vi "myRIO_BRig_FPGA_v3,50.vi"() -> ()   [LabVIEW 2014]
uses:
  <vilib>/rvi/FXPMathLib/FxpMul/XNode/nifxpmath_Multiplier.xnode
  <vilib>/rvi/FXPMathLib/sim/FxpSim.dll
  <vilib>/eio/EIONode/EIONode.xnode
  <vilib>/rvi/eio/common/nirviEmuTemplateMethod_errors.vi
panel:
  in  "k1__counter_per_ms":u16=100 min=100 max=40000 step=1
  in  "laser_Nshutter":u32=100
  in  "AnaOut_0":u16
  in  "laser_Nvalley":u32=100
  in  "laser_Npeak":u32=100
  in  "laserledMTrig":bool
  in  "laser_selWro_Ntotal":u32=100
  in  "laser_selWro_NDelay":u32
  in  "laser_selRew_Ntotal":u32=100
  in  "laser_selRew_Ndelay":u32
  in  "laserResponse_reward_LED":bool
  in  "laserResponse_wrong_LED":bool
  out "SelectWrong":bool
  out "SelectReward":bool
  in  "laserResponse_wrong":bool
  in  "laserResponse_reward":bool
  in  "Left(F)_or_Right(T)":bool
  in  "ignoreWrong":bool
  in  "SelectionState":bool
  in  "laserMTrig":bool
  in  "FPGA_Stop":bool
  in  "audioTrigger_L":bool
  in  "audioTrigger_R":bool
  in  "audioFreq_L_kHz":u8=14 min=1 max=14 step=1
  in  "audioAmp_L":u16=1 min=1 max=32767 step=1
  in  "audioFreq_R_kHz":u8=14 min=1 max=14 step=1
  in  "audioAmp_R":u16=1 min=1 max=32767 step=1
  in  "A3_SL":bool
  in  "A1_SR":bool
  in  "Counts_Reset":bool
  out "A4_LickR":u32
  out "A2_LickL":u32
  in  "A6_Act":bool
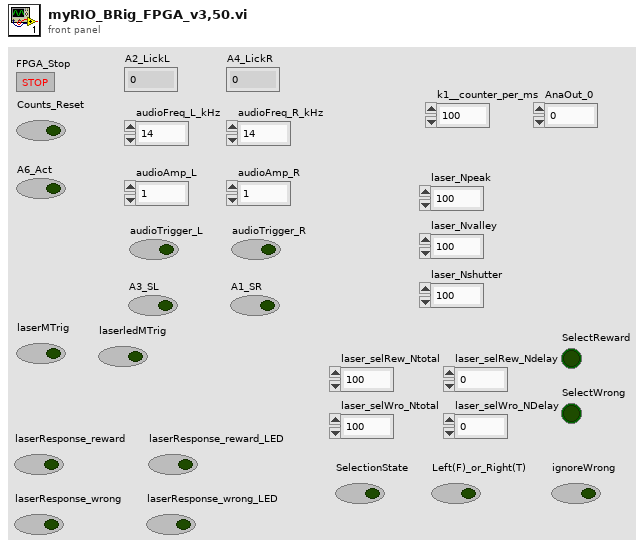
[diagram p1: front panel]
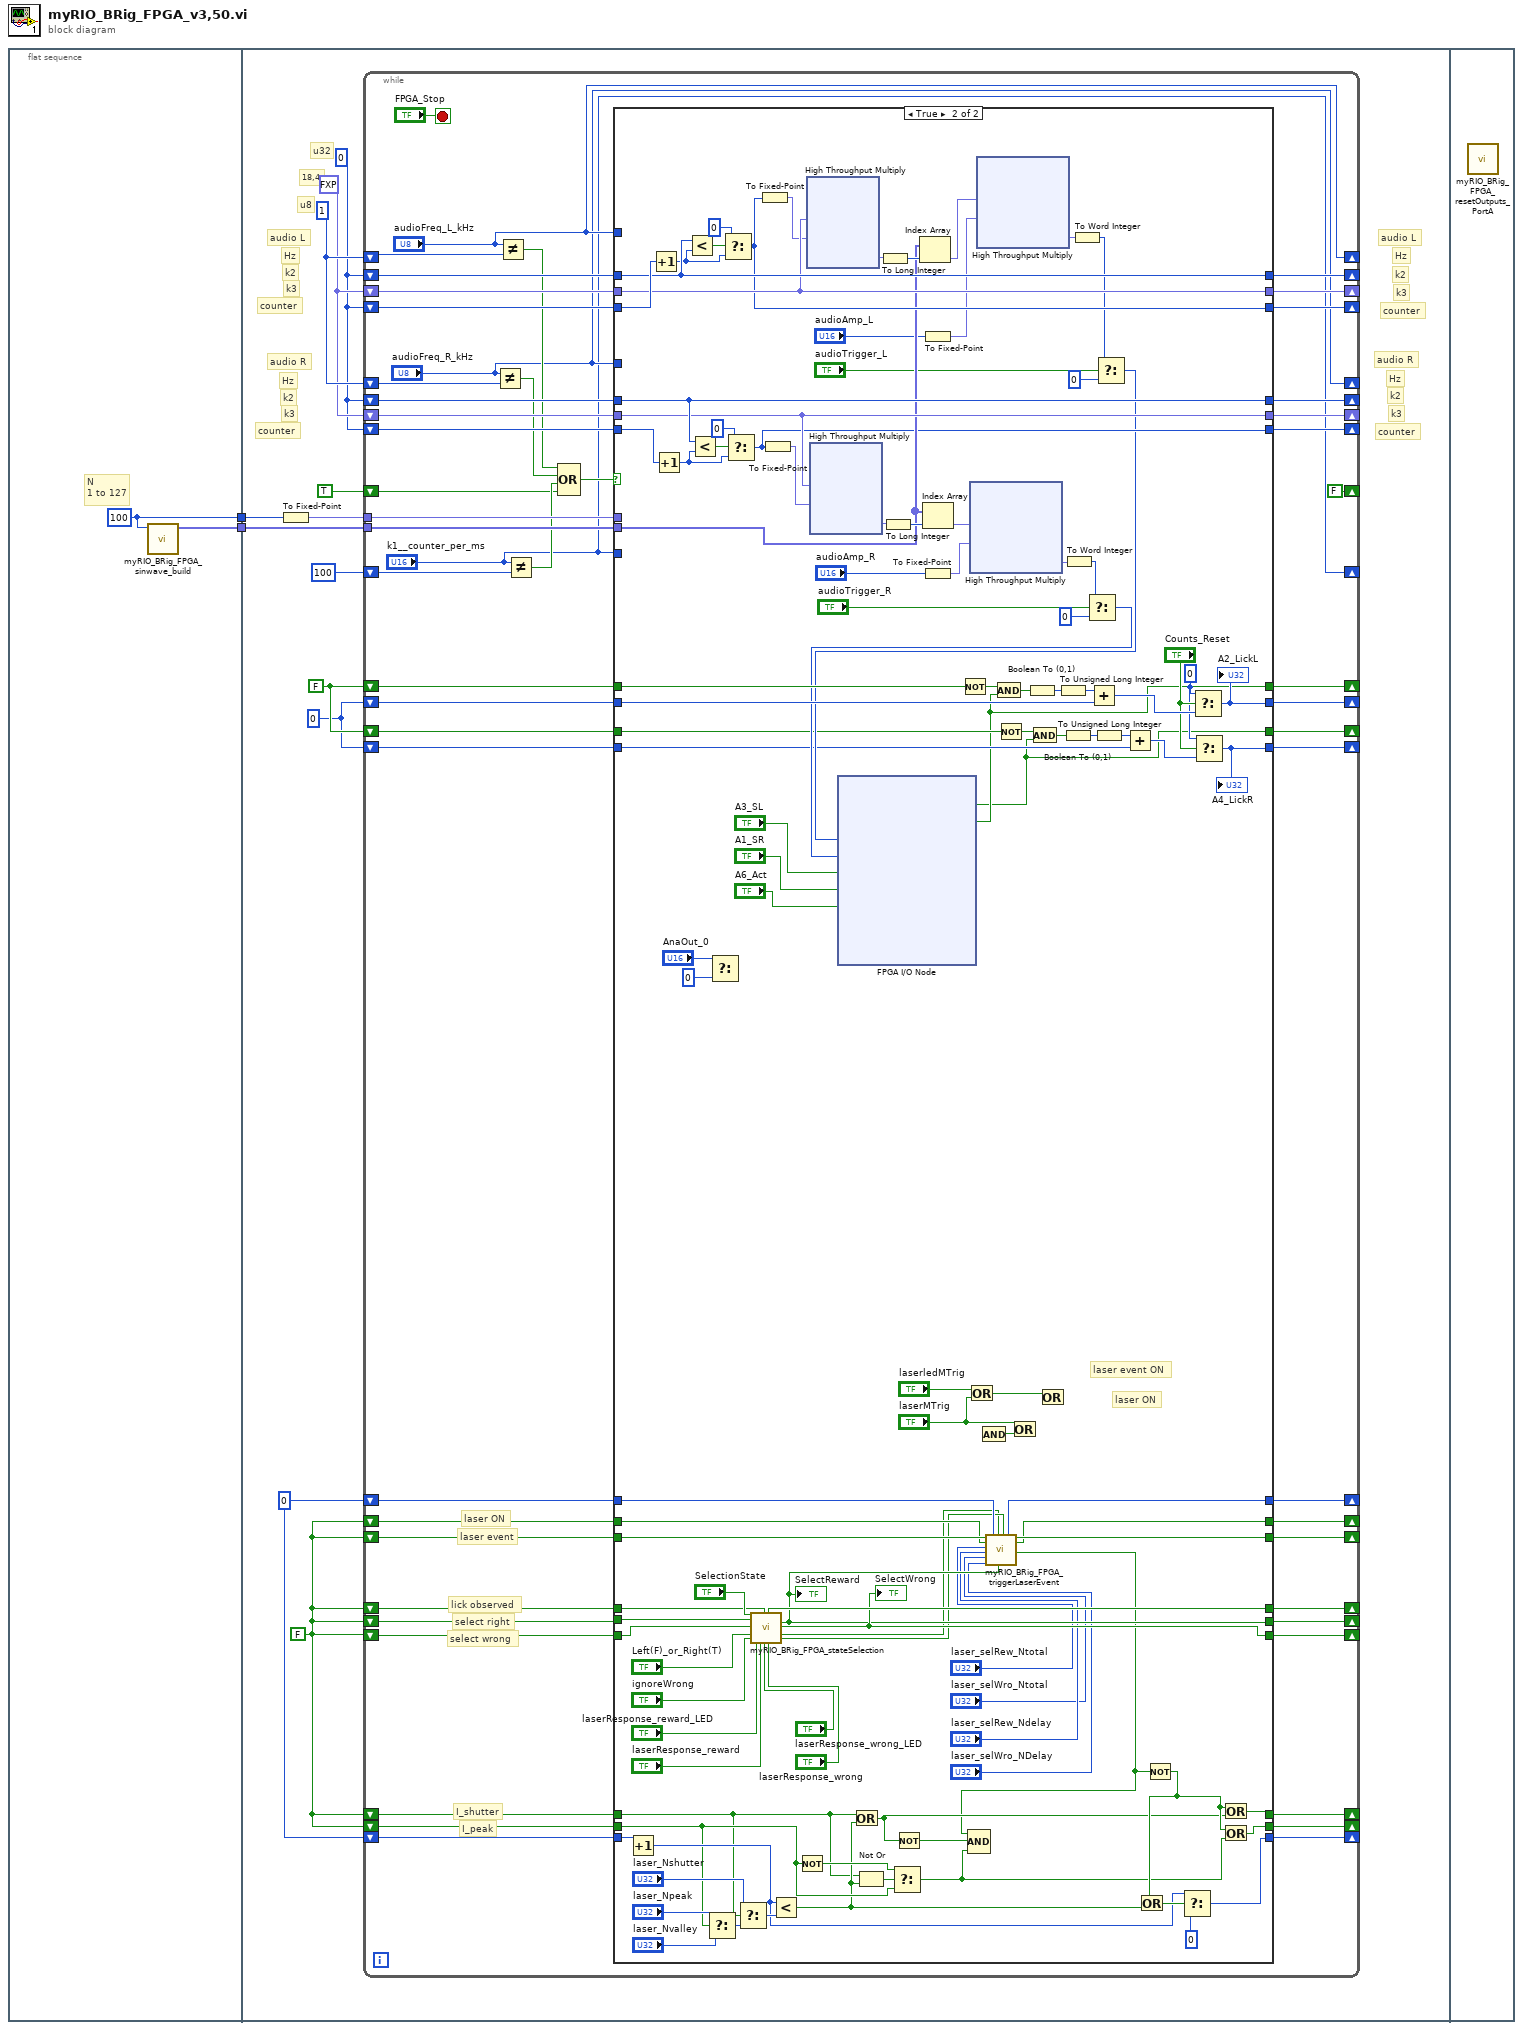
[diagram p0: block diagram]
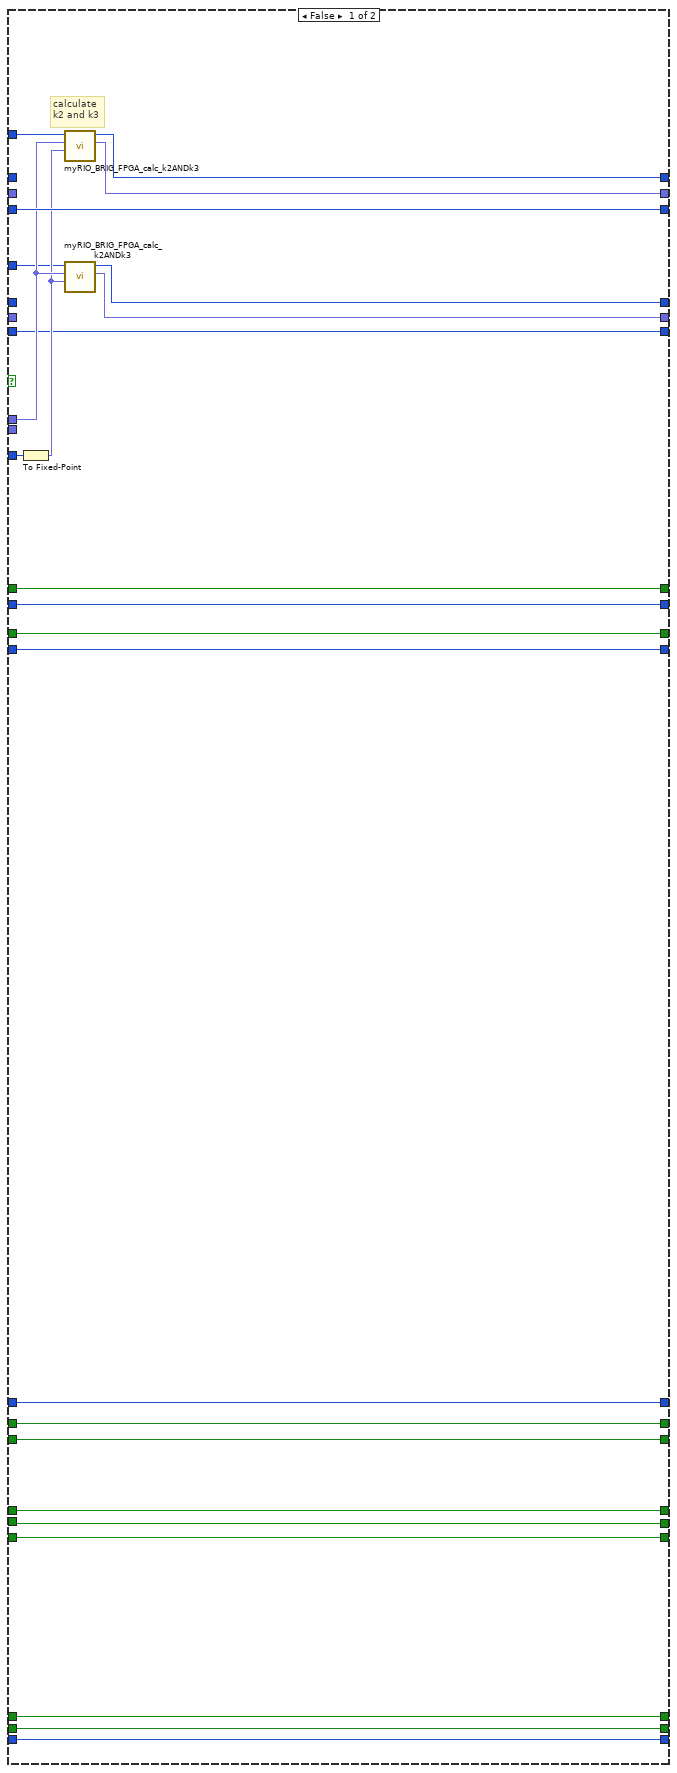
[diagram p2: hidden frame]
diagram:
  n1 = flat-sequence {
    tunnel: [w4] -> w2
    tunnel: [w3] -> w1
    tunnel: w2 -> [w16]
    tunnel: w1 -> [w15]
    frame #0 {
      w3 = 100 ("dimension size")
      # "N\n1 to 127"
      n2 = call "myRIO_BRig_FPGA_sinwave_build.vi"("input_Npts"=w3) -> ("output_array_sin"=w4:fxp<+/-,16,2>[])  [unwired: 10 in]
    }
    frame #1 {
      w5 = u32 0
      w6 = FALSE
      w7 = u32 0
      w8 = FALSE
      w11 = u32 0
      w12 = fxp<+,18,4> 0.0
      w13 = u8 1
      # "counter"
      # "k3"
      # "k2"
      # "counter"
      # "k3"
      # "k2"
      # "counter"
      # "counter"
      # "u32"
      # "k3"
      # "k2"
      # "k3"
      # "18,4"
      # "u8"
      # "Hz"
      # "Hz"
      # "audio R"
      # "audio L"
      # "Hz"
      # "k2"
      # "Hz"
      # "audio R"
      # "audio L"
      n3 = To Fixed-Point(number=w15) -> (fixed-point=w14:fxp<+,7,7>)  [unwired: 1 in]
      n4 = while {
        shift-right: ["audioFreq_L_kHz"] -> _
        shift-left: w13 -> [w69]
        shift-right: [w63] -> _
        shift-left: w11 -> [w67]
        shift-right: ["audioFreq_R_kHz"] -> _
        shift-left: w13 -> [w59]
        tunnel: w16 -> [w66]
        tunnel: w14 -> [w65]
        shift-right: [w62] -> _
        shift-left: w12 -> [w64]
        shift-right: [w60] -> _
        shift-left: w11 -> [w61]
        shift-right: [w57] -> _
        shift-left: w11 -> [w58]
        shift-right: [w55] -> _
        shift-left: w12 -> [w56]
        shift-right: [w53] -> _
        shift-left: w11 -> [w54]
        shift-right: ["k1__counter_per_ms"] -> _
        shift-left: u16 100 ("y") -> [w52]
        shift-right: [FALSE] -> _
        shift-left: TRUE -> [w47]
        shift-right: [w40] -> _
        shift-left: w8 -> [w42]
        shift-right: [w39] -> _
        shift-left: w8 -> [w41]
        shift-right: [w37] -> _
        shift-left: w7 -> [w38]
        shift-right: [w35] -> _
        shift-left: w7 -> [w36]
        shift-right: [w33] -> _
        shift-left: w6 -> [w34]
        shift-right: [w30] -> _
        shift-left: w6 -> [w32]
        shift-right: [w29] -> _
        shift-left: w6 -> [w31]
        shift-right: [w26] -> _
        shift-left: w6 -> [w25]
        shift-right: [w27] -> _
        shift-left: w6 -> [w28]
        shift-right: [w23] -> _
        shift-left: w5 -> [w24]
        shift-right: [w19] -> _
        shift-left: w6 -> [w22]
        shift-right: [w18] -> _
        shift-left: w6 -> [w21]
        shift-right: [w17] -> _
        shift-left: w5 -> [w20]
        stop <- "FPGA_Stop" stop-if-true
        # "I_shutter"
        # "I_peak"
        # "laser ON"
        # "laser event"
        # "select wrong"
        # "select right"
        # "lick observed"
        n5 = Not Equal?(x="audioFreq_R_kHz", y=w59) -> (x != y?=w50:bool)
        n6 = Not Equal?(x="audioFreq_L_kHz", y=w69) -> (x != y?=w51:bool)
        n7 = Not Equal?(x="k1__counter_per_ms", y=w52) -> (x != y?=w48:bool)
        n8 = Compound Arithmetic op=OR(w51, w50, w48, w47) -> (w49:bool)
        n9 = case shown="True" w49 {
          tunnel: w67 -> [_ w205]
          tunnel: "audioFreq_L_kHz" -> [w92 _]
          tunnel: w66 -> [_ w187]
          tunnel: w65 -> [w88 _]
          tunnel: "k1__counter_per_ms" -> [w93 _]
          tunnel: w64 -> [_ w201]
          tunnel: [w91 w205] -> w63
          tunnel: [w90 w201] -> w62
          tunnel: w61 -> [w89 w206]
          tunnel: [w89 w197] -> w60
          tunnel: w58 -> [_ w191]
          tunnel: [w84 w191] -> w57
          tunnel: w56 -> [_ w188]
          tunnel: [w85 w188] -> w55
          tunnel: w54 -> [w83 w190]
          tunnel: "audioFreq_R_kHz" -> [w86 _]
          tunnel: [w83 w186] -> w53
          tunnel: w42 -> [w82 w169]
          tunnel: w41 -> [w81 w157]
          tunnel: [w82 w143] -> w40
          tunnel: [w81 w142] -> w39
          tunnel: w38 -> [w80 w167]
          tunnel: [w80 w164] -> w37
          tunnel: w36 -> [w79 w156]
          tunnel: [w79 w152] -> w35
          tunnel: w34 -> [w78 w145]
          tunnel: [w78 w144] -> w33
          tunnel: w32 -> [w77 w147]
          tunnel: w31 -> [w76 w146]
          tunnel: [w77 w128] -> w30
          tunnel: [w76 w135] -> w29
          tunnel: w28 -> [w75 w133]
          tunnel: [w75 w129] -> w27
          tunnel: [w74 w130] -> w26
          tunnel: w25 -> [w74 w134]
          tunnel: w24 -> [w73 w132]
          tunnel: [w73 w131] -> w23
          tunnel: w22 -> [w72 w104]
          tunnel: w21 -> [w71 w109]
          tunnel: w20 -> [w70 w121]
          tunnel: [w72 w106] -> w19
          tunnel: [w71 w108] -> w18
          tunnel: [w70 w112] -> w17
          frame False {
            # "calculate\nk2 and k3"
            n10 = To Fixed-Point(number=w93) -> (fixed-point=w87:fxp<+,16,16>)  [unwired: 1 in]
            n11 = call "myRIO_BRIG_FPGA_calc_k2ANDk3.vi"("input_k1[count/ms]"=w87, "input_Npts"=w88, "input_freq[kHz]"=w92) -> ("output_k3"=w90:fxp<+,18,4>, "output_k2"=w91:u32)  [unwired: 7 in]
            n12 = call "myRIO_BRIG_FPGA_calc_k2ANDk3.vi"("input_k1[count/ms]"=w87, "input_Npts"=w88, "input_freq[kHz]"=w86) -> ("output_k3"=w85:fxp<+,18,4>, "output_k2"=w84:u32)  [unwired: 7 in]
          }
          frame True {
            w154 = u32 0 ("t")
            # "laser ON"
            # "laser event ON"
            n13 = Increment(x=w121) -> (x+1=w113:u32)
            n14 = Increment(x=w206) -> (x+1=w203:u32)
            n15 = Increment(x=w190) -> (x+1=w189:u32)
            n16 = Less?(x=w205, y=w203) -> (x < y?=w204:bool)
            n17 = Less?(x=w191, y=w189) -> (x < y?=w196:bool)
            n18 = Select(t="laser_Npeak", s=w109, f="laser_Nvalley") -> (s? t:f=w120:u32)
            n19 = Select(t="AnaOut_0", f=u16 0) -> ()  [unwired: 1 in, 1 out]
            n20 = Select(t=u32 0, s=w204, f=w203) -> (s? t:f=w197:u32)
            n21 = Select(t=u32 0, s=w196, f=w189) -> (s? t:f=w186:u32)
            n22 = Select(t="laser_Nshutter", s=w104, f=w120) -> (s? t:f=w116:u32)
            n23 = call "myRIO_BRig_FPGA_stateSelection.vi"("I_selectionState"="SelectionState", "I_selectRight"=w147, "I_selectWrong"=w146, "I_Left(F)_or_Right(T)"="Left(F)_or_Right(T)", "I_ignoreWrong"="ignoreWrong", "I_laserEvent_Reward"="laserResponse_reward_LED", "I_laser_Reward"="laserResponse_reward", "I_lickObserved"=w145, "I_laserEvent_Wrong"="laserResponse_wrong_LED", "I_laser_Wrong"="laserResponse_wrong") -> ("output_I_lickObserved"=w144:bool, "output__I_selectRight"=w128:bool, "output__I_selectWrong"=w135:bool, "output_I_startLaserEvent"=w94:bool, "output_I_startLaser"=w95:bool)  [unwired: 13 in]
            "SelectWrong" <- w135
            "SelectReward" <- w128
            n24 = To Fixed-Point(number=w197) -> (fixed-point=w200:fxp<+,32,32>)  [unwired: 1 in]
            n25 = To Fixed-Point(number=w186) -> (fixed-point=w194:fxp<+,32,32>)  [unwired: 1 in]
            n26 = Less?(x=w113, y=w116) -> (x < y?=w105:bool)
            n27 = Not(x=w109) -> (.not. x?=w110:bool)
            n28 = xnode "High Throughput Multiply"("x"=w201, "y"=w200) -> ("x*y"=w199:fxp<+,7,7>)
            n29 = xnode "High Throughput Multiply"("x"=w188, "y"=w194) -> ("x*y"=w193:fxp<+,7,7>)
            n30 = Or(x=w104, y=w105) -> (x .or. y?=w103:bool)
            n31 = Not Or(1:w105, 2:w104) -> (0:w111:bool)
            n32 = To Long Integer(number=w199) -> (32bit integer=w198:i32)
            n33 = To Long Integer(number=w193) -> (32bit integer=w192:i32)
            n34 = Select(t=w110, s=w111, f=w109) -> (s? t:f=w101:bool)
            n35 = Not(x=w103) -> (.not. x?=w102:bool)
            n36 = Index Array(array=w187, index=w198) -> (element=w174:fxp<+/-,16,2>)
            n37 = To Fixed-Point(number="audioAmp_L") -> (fixed-point=w177:fxp<+,15,15>)  [unwired: 1 in]
            n38 = Index Array(array=w187, index=w192) -> (element=w184:fxp<+/-,16,2>)
            n39 = To Fixed-Point(number="audioAmp_R") -> (fixed-point=w182:fxp<+,15,15>)  [unwired: 1 in]
            n40 = Not(x=w169) -> (.not. x?=w166:bool)
            n41 = Or(x="laserledMTrig", y="laserMTrig") -> (x .or. y?=w98:bool)
            n42 = xnode ("High Throughput Multiply")("x"=w184, "y"=w182) -> ("x*y"=w185:fxp<+/-,31,17>)
            n43 = xnode ("High Throughput Multiply")("x"=w174, "y"=w177) -> ("x*y"=w178:fxp<+/-,31,17>)
            n44 = And() -> (x .and. y?=w97:bool)  [unwired: 2 in]
            n45 = call "myRIO_BRig_FPGA_triggerLaserEvent.vi"("I_laserEvent"=w134, "I_laser"=w133, "laser_selRew_Ntotal"="laser_selRew_Ntotal", "laser_selRew_Ndelay"="laser_selRew_Ndelay", "laser_selWro_Ntotal"="laser_selWro_Ntotal", "laser_selWro_NDelay"="laser_selWro_NDelay", "counter"=w132, "I_startLaserEvent"=w94, "selectReward"=w128, "I_startLaser"=w95) -> ("output_counter"=w131:u32, "output_I_laserEvent"=w130:bool, "output_I_laser"=w129:bool, "output_I_trigLaserEvent"=w100:bool)  [unwired: 5 in, 1 out]
            n46 = Compound Arithmetic op=AND(w100, w102, w101) -> ()  [unwired: 1 out]
            n47 = Not(x=w157) -> (.not. x?=w158:bool)
            n48 = Or(x="laserMTrig", y=w97) -> ()  [unwired: 1 out]
            n49 = Or(x=w98) -> ()  [unwired: 1 in, 1 out]
            n50 = To Word Integer(number=w185) -> (16bit integer=w180:i16)
            n51 = To Word Integer(number=w178) -> (16bit integer=w176:i16)
            n52 = Select(t=w180, s="audioTrigger_R", f=i16 0) -> (s? t:f=w163:i16)
            n53 = Select(t=w176, s="audioTrigger_L", f=i16 0) -> (s? t:f=w162:i16)
            n54 = xnode "FPGA I/O Node"("AudioOut/Left"=w162, "AudioOut/Right"=w163, "ConnectorA/DIO3"="A3_SL", "ConnectorA/DIO1"="A1_SR", "ConnectorA/DIO7"="A6_Act") -> ("ConnectorA/DIO4"=w142:bool, "ConnectorA/DIO2"=w143:bool)  [unwired: 13 in, 10 out]
            n55 = And(x=w166, y=w143) -> (x .and. y?=w170:bool)
            n56 = Boolean To (0,1)(Boolean=w170) -> (0, 1=w171:i16)
            n57 = And(x=w158, y=w142) -> (x .and. y?=w160:bool)
            n58 = To Unsigned Long Integer(number=w171) -> (unsigned 32bit integer=w168:u32)
            n59 = Boolean To (0,1)(Boolean=w160) -> (0, 1=w161:i16)
            n60 = Add(x=w168, y=w167) -> (x+y=w165:u32)
            n61 = To Unsigned Long Integer(number=w161) -> (unsigned 32bit integer=w159:u32)
            n62 = Add(x=w159, y=w156) -> (x+y=w153:u32)
            n63 = Not(x=w100) -> (.not. x?=w107:bool)
            n64 = Or(x=w107, y=w105) -> (x .or. y?=w114:bool)
            n65 = Select(t=w113, s=w114, f=u32 0) -> (s? t:f=w112:u32)
            n66 = Select(t=w154, s="Counts_Reset", f=w165) -> (s? t:f=w164:u32)
            "A2_LickL" <- w164
            n67 = Select(t=w154, s="Counts_Reset", f=w153) -> (s? t:f=w152:u32)
            "A4_LickR" <- w152
            n68 = Or(x=w107, y=w103) -> (x .or. y?=w106:bool)
            n69 = Or(x=w107, y=w101) -> (x .or. y?=w108:bool)
          }
        }
      }
    }
    frame #2 {
      n70 = call "myRIO_BRig_FPGA_resetOutputs_PortA.vi"() -> ()  [unwired: 12 in]
    }
  }
